vi "oscCtrlDemo.vi"() -> ()   [LabVIEW 2016]
panel:
  in  "Send":string
  in  "send Button":bool
  in  "query Button":bool
  out "read buffer":string
  in  "Query String":string
  in  "VISA resource name":refnum<visa-resource-name>
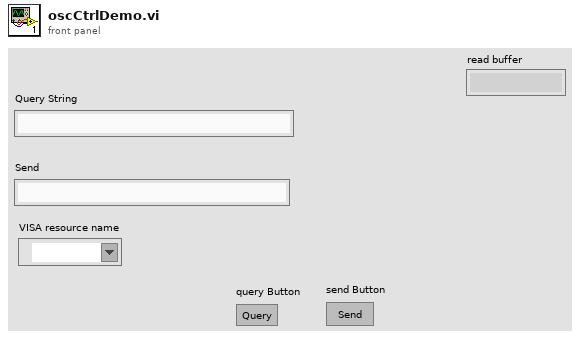
[diagram p1: front panel]
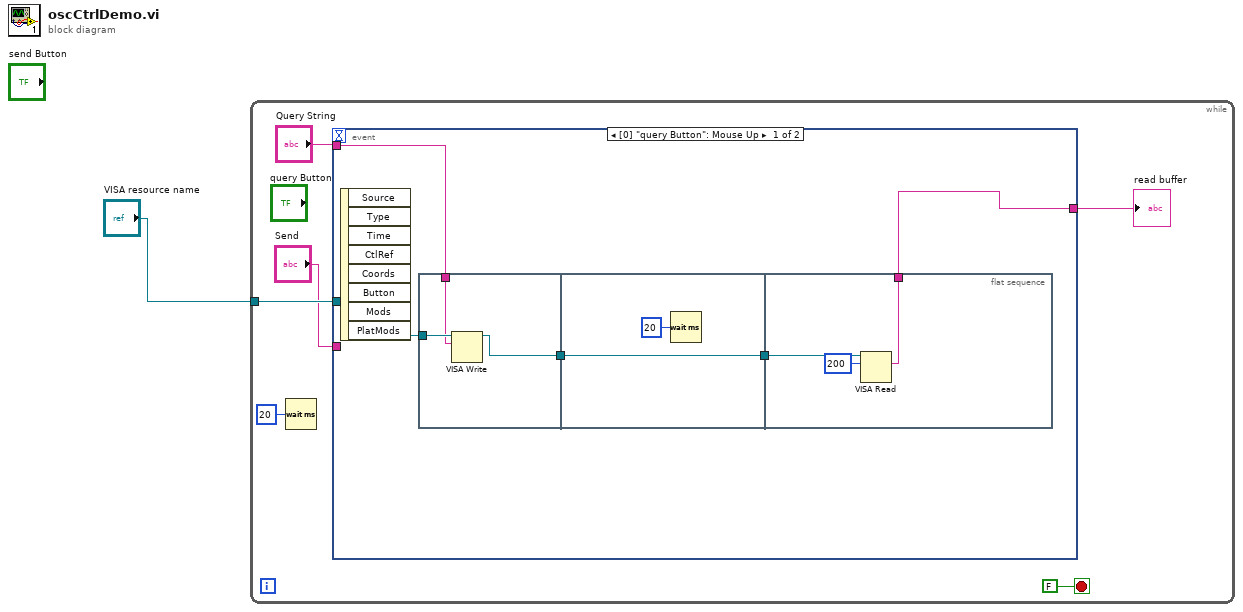
[diagram p0: block diagram]
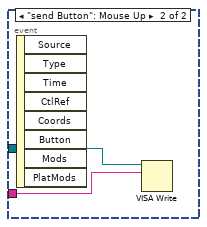
[diagram p2: hidden frame]
diagram:
  n1 = while {
    tunnel: "VISA resource name" -> [w7]
    stop <- FALSE stop-if-true
    n2 = Wait (ms)(milliseconds to wait=u32 20) -> ()  [unwired: 1 out]
    n3 = event shown="[0] \"query Button\": Mouse Up" {
      selector: _ -> [_ _]
      dyn-events: _ -> [_ _]
      timeout: _ -> [_ _]
      tunnel: w7 -> [w10 w22]
      tunnel: "Query String" -> [w9 _]
      tunnel: "Send" -> [_ w21]
      tunnel: [w8 _] -> w2
      event "query Button": Mouse Up {
        n4 = event-data() -> ()  [unwired: 1 in, 8 out]
        n5 = flat-sequence {
          tunnel: w10 -> [w15]
          tunnel: w9 -> [w14]
          tunnel: [w13] -> w12
          tunnel: [w17] -> w11
          tunnel: w12 -> [w17]
          tunnel: w11 -> [w20]
          tunnel: [w19] -> w8
          frame #0 {
            n6 = VISA Write(VISA resource name=w15, write buffer=w14) -> (VISA resource name out=w13:refnum<visa-resource-name>)  [unwired: 1 in, 2 out]
          }
          frame #1 {
            n7 = Wait (ms)(milliseconds to wait=u32 20) -> ()  [unwired: 1 out]
          }
          frame #2 {
            n8 = VISA Read(VISA resource name=w20, byte count=u32 200) -> (read buffer=w19:string)  [unwired: 1 in, 3 out]
          }
        }
      }
      event "send Button": Mouse Up {
        n9 = event-data() -> ()  [unwired: 1 in, 8 out]
        n10 = VISA Write(VISA resource name=w22, write buffer=w21) -> ()  [unwired: 1 in, 3 out]
      }
    }
    "read buffer" <- w2
  }
